vi "RenameTerminals.vi"(6 "Dynamic Dispatch":bool, 8 "error in (no error)":errorcluster, 11 "CreateClass In":refnum<class "CreateClass.lvclass">) -> (0 "error out":errorcluster)   [LabVIEW 2020, in "Mermaid.lvlib" / "CreateClass.lvclass"]
uses:
  CreateClass.lvclass
  CreateClass.lvclass/CreateClass.ctl
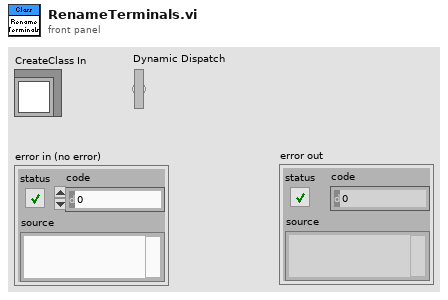
[diagram p1: front panel]
types:
  T1 = enum16{"Invalid Wire Rule", "Required", "Recommended", "Optional", "Dynamic Dispatch"}
  T2 = enum16{"Invalid Wire Rule", "Required", "Recommended", "Optional", "Dynamic Dispatch"}[]
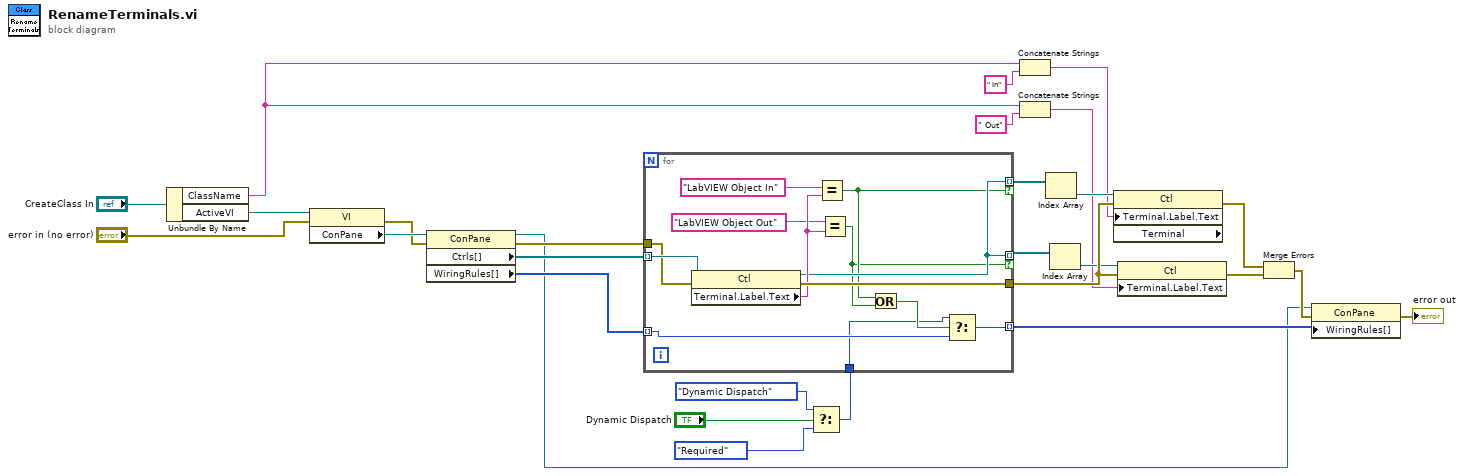
[diagram p0: block diagram]
diagram:
  n1 = Unbundle By Name("CreateClass In") -> ("ClassName"=w7:string, "ActiveVI"=w26:refnum<vi>)
  n2 = property class="VI"(reference=w26, error in="error in (no error)") -> (error out=w12:errorcluster, "ConPane"=w22:refnum<vi>)  [unwired: 1 out]
  n3 = property class="ConPane"(reference=w22, error in=w12) -> (reference out=w2:refnum<vi>, error out=w14:errorcluster, "Ctrls[]"=w13:refnum<vi>[], "WiringRules[]"=w23:T2)
  n4 = Select(t=T1."Dynamic Dispatch" ("Wire Rule"), s="Dynamic Dispatch", f=T1."Required" ("Wire Rule")) -> (s? t:f=w3:T1)
  n5 = for {
    tunnel: w13 -> [w41] mode=indexing
    tunnel: w14 -> [w40]
    tunnel: [w39] -> w19
    tunnel: [w35] -> w15 mode=indexing if=w34
    tunnel: [w35] -> w18 mode=indexing if=w33
    tunnel: w23 -> [w31] mode=indexing
    tunnel: [w30] -> w25 mode=indexing
    tunnel: w3 -> [w29]
    n6 = property class="Ctl"(reference=w41, error in=w40) -> (reference out=w35:refnum<vi>, error out=w39:errorcluster, "Terminal.Label.Text"=w38:string)
    n7 = Equal?(x="LabVIEW Object In" ("name/order"), y=w38) -> (x = y?=w34:bool)
    n8 = Equal?(x="LabVIEW Object Out" ("name/order"), y=w38) -> (x = y?=w33:bool)
    n9 = Or(x=w34, y=w33) -> (x .or. y?=w32:bool)
    n10 = Select(t=w29, s=w32, f=w31) -> (s? t:f=w30:T1)
  }
  n11 = Concatenate Strings(w7, " In" ("string")) -> (w9:string)
  n12 = Concatenate Strings(w7, " Out" ("string")) -> (w8:string)
  n13 = Index Array(array=w15) -> (element=w16:refnum<vi>)  [unwired: 1 in]
  n14 = Index Array(array=w18) -> (element=w17:refnum<vi>)  [unwired: 1 in]
  n15 = property class="Ctl" props=["Terminal", "Label", "Text", "Terminal"](reference=w16, error in=w19, "Terminal.Label.Text"=w9) -> (error out=w21:errorcluster)  [unwired: 2 out]
  n16 = property class="Ctl"(reference=w17, error in=w19, "Terminal.Label.Text"=w8) -> (error out=w20:errorcluster)  [unwired: 1 out]
  n17 = Merge Errors(w21, w20) -> (w24:errorcluster)
  n18 = property class="ConPane"(reference=w2, error in=w24, "WiringRules[]"=w25) -> (error out=→"error out":errorcluster)  [unwired: 1 out]
